vi "Configure Measurement.vi"(8 "error in (no error)":errorcluster, 9 "function (Z - Angle:0)":u16(ring) items=["Z - Angle", "R - X", "Y - Angle", "G - B", "CP - D", "CP - Q", "CP - G", "CS - D", "CS - Q", "CS - RS", "LP - D", "LP - Q", "LP - G", "LS - D", "LS - Q", "LS - RS", "LS - DCR (option 001 only)", "LP - DCR (option 001 only)", "L2 - N (option 001 only)", "L2 - M (option 001 only)", "L2 - R2 (option 001 only)"], 11 "VISA resource name":refnum<visa-resource-name>) -> (0 "error out":errorcluster, 3 "VISA resource name out":refnum<visa-resource-name>)   [LabVIEW 2016, in "Agilent 4263X.lvlib"]
doc: "This VI configures the primary and secondary measurement combinations which can be taken by the instrument."
uses:
  <instrlib>/Agilent 4263X/Agilent 4263X.lvlib
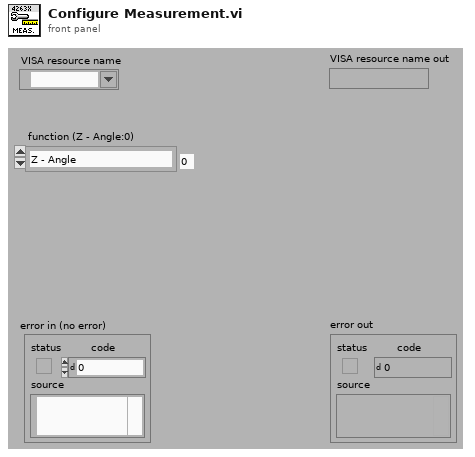
[diagram p1: front panel]
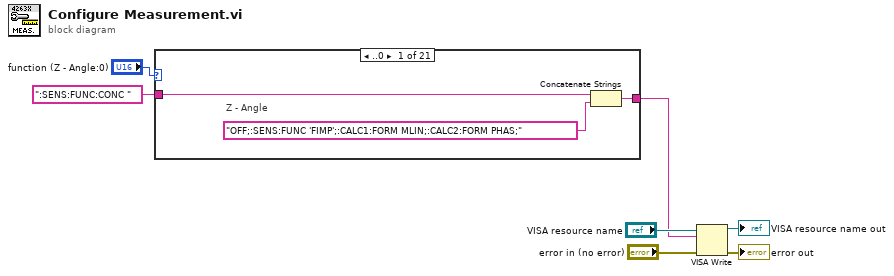
[diagram p0: block diagram]
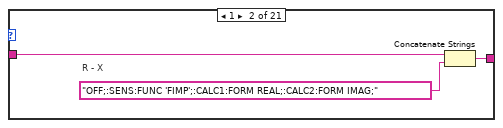
[diagram p2: hidden frame]
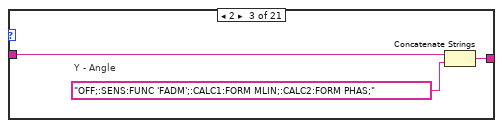
[diagram p3: hidden frame]
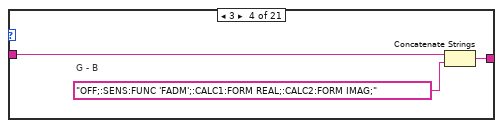
[diagram p4: hidden frame]
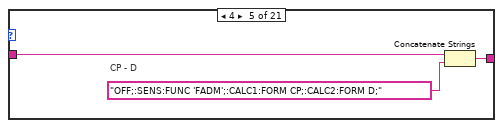
[diagram p5: hidden frame]
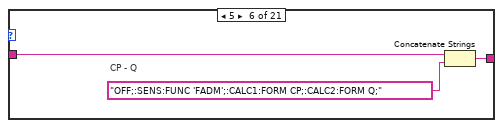
[diagram p6: hidden frame]
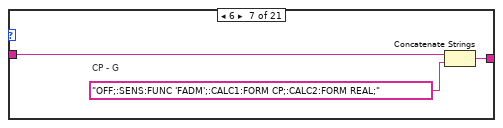
[diagram p7: hidden frame]
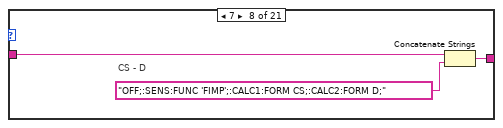
[diagram p8: hidden frame]
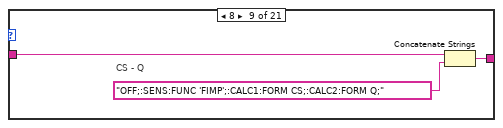
[diagram p9: hidden frame]
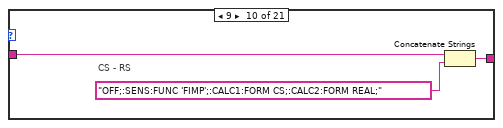
[diagram p10: hidden frame]
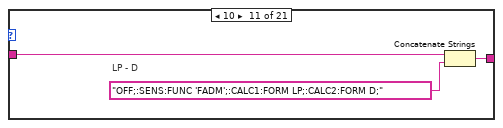
[diagram p11: hidden frame]
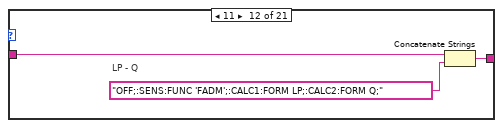
[diagram p12: hidden frame]
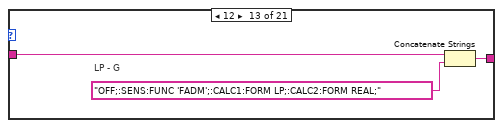
[diagram p13: hidden frame]
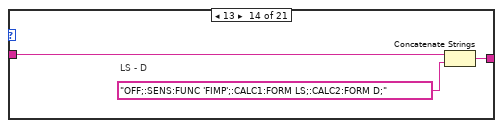
[diagram p14: hidden frame]
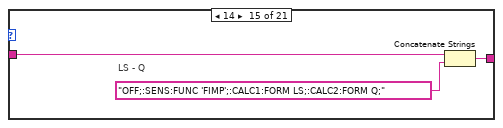
[diagram p15: hidden frame]
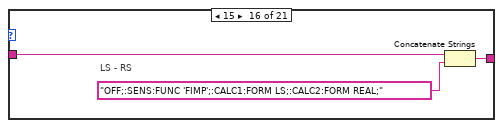
[diagram p16: hidden frame]
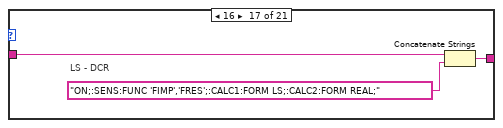
[diagram p17: hidden frame]
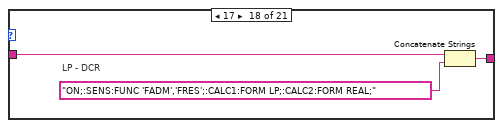
[diagram p18: hidden frame]
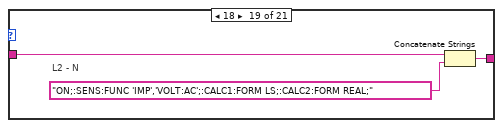
[diagram p19: hidden frame]
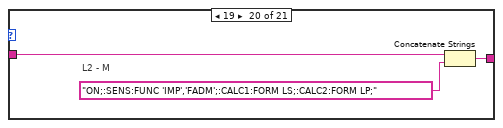
[diagram p20: hidden frame]
diagram:
  n1 = case shown="..0" "function (Z - Angle:0)" {
    tunnel: ":SENS:FUNC:CONC " -> [w10 w13 w16 w19 w22 w25 w28 w31 w34 w37 w40 w43 w46 w49 w52 w55 w58 w61 w64 w67 w70]
    tunnel: [w8 w11 w14 w17 w20 w23 w26 w29 w32 w35 w38 w41 w44 w47 w50 w53 w56 w59 w62 w65 w68] -> w1
    frame ..0 {
      # "Z - Angle"
      n2 = Concatenate Strings(w10, "OFF;:SENS:FUNC 'FIMP';:CALC1:FORM MLIN;:CALC2:FORM PHAS;") -> (w8:string)
    }
    frame 1 {
      # "R - X"
      n3 = Concatenate Strings(w13, "OFF;:SENS:FUNC 'FIMP';:CALC1:FORM REAL;:CALC2:FORM IMAG;") -> (w11:string)
    }
    frame 2 {
      # "Y - Angle"
      n4 = Concatenate Strings(w16, "OFF;:SENS:FUNC 'FADM';:CALC1:FORM MLIN;:CALC2:FORM PHAS;") -> (w14:string)
    }
    frame 3 {
      # "G - B"
      n5 = Concatenate Strings(w19, "OFF;:SENS:FUNC 'FADM';:CALC1:FORM REAL;:CALC2:FORM IMAG;") -> (w17:string)
    }
    frame 4 {
      # "CP - D"
      n6 = Concatenate Strings(w22, "OFF;:SENS:FUNC 'FADM';:CALC1:FORM CP;:CALC2:FORM D;") -> (w20:string)
    }
    frame 5 {
      # "CP - Q"
      n7 = Concatenate Strings(w25, "OFF;:SENS:FUNC 'FADM';:CALC1:FORM CP;:CALC2:FORM Q;") -> (w23:string)
    }
    frame 6 {
      # "CP - G"
      n8 = Concatenate Strings(w28, "OFF;:SENS:FUNC 'FADM';:CALC1:FORM CP;:CALC2:FORM REAL;") -> (w26:string)
    }
    frame 7 {
      # "CS - D"
      n9 = Concatenate Strings(w31, "OFF;:SENS:FUNC 'FIMP';:CALC1:FORM CS;:CALC2:FORM D;") -> (w29:string)
    }
    frame 8 {
      # "CS - Q"
      n10 = Concatenate Strings(w34, "OFF;:SENS:FUNC 'FIMP';:CALC1:FORM CS;:CALC2:FORM Q;") -> (w32:string)
    }
    frame 9 {
      # "CS - RS"
      n11 = Concatenate Strings(w37, "OFF;:SENS:FUNC 'FIMP';:CALC1:FORM CS;:CALC2:FORM REAL;") -> (w35:string)
    }
    frame 10 {
      # "LP - D"
      n12 = Concatenate Strings(w40, "OFF;:SENS:FUNC 'FADM';:CALC1:FORM LP;:CALC2:FORM D;") -> (w38:string)
    }
    frame 11 {
      # "LP - Q"
      n13 = Concatenate Strings(w43, "OFF;:SENS:FUNC 'FADM';:CALC1:FORM LP;:CALC2:FORM Q;") -> (w41:string)
    }
    frame 12 {
      # "LP - G"
      n14 = Concatenate Strings(w46, "OFF;:SENS:FUNC 'FADM';:CALC1:FORM LP;:CALC2:FORM REAL;") -> (w44:string)
    }
    frame 13 {
      # "LS - D"
      n15 = Concatenate Strings(w49, "OFF;:SENS:FUNC 'FIMP';:CALC1:FORM LS;:CALC2:FORM D;") -> (w47:string)
    }
    frame 14 {
      # "LS - Q"
      n16 = Concatenate Strings(w52, "OFF;:SENS:FUNC 'FIMP';:CALC1:FORM LS;:CALC2:FORM Q;") -> (w50:string)
    }
    frame 15 {
      # "LS - RS"
      n17 = Concatenate Strings(w55, "OFF;:SENS:FUNC 'FIMP';:CALC1:FORM LS;:CALC2:FORM REAL;") -> (w53:string)
    }
    frame 16 {
      # "LS - DCR"
      n18 = Concatenate Strings(w58, "ON;:SENS:FUNC 'FIMP','FRES';:CALC1:FORM LS;:CALC2:FORM REAL;") -> (w56:string)
    }
    frame 17 {
      # "LP - DCR"
      n19 = Concatenate Strings(w61, "ON;:SENS:FUNC 'FADM','FRES';:CALC1:FORM LP;:CALC2:FORM REAL;") -> (w59:string)
    }
    frame 18 {
      # "L2 - N"
      n20 = Concatenate Strings(w64, "ON;:SENS:FUNC 'IMP','VOLT:AC';:CALC1:FORM LS;:CALC2:FORM REAL;") -> (w62:string)
    }
    frame 19 {
      # "L2 - M"
      n21 = Concatenate Strings(w67, "ON;:SENS:FUNC 'IMP','FADM';:CALC1:FORM LS;:CALC2:FORM LP;") -> (w65:string)
    }
    frame 20.. {
      # "L2 - R2"
      n22 = Concatenate Strings(w70, "ON;:SENS:FUNC 'IMP','RES';:CALC1:FORM LS;:CALC2:FORM REAL;") -> (w68:string)
    }
  }
  n23 = VISA Write(VISA resource name="VISA resource name", write buffer=w1, error in (no error)="error in (no error)") -> (VISA resource name out=→"VISA resource name out":refnum<visa-resource-name>, error out=→"error out":errorcluster)  [unwired: 1 out]
